vi "7 - Dynamically Rebind Event Handlers.vi"() -> ()   [LabVIEW 2012]
panel:
  out "Slide":dbl(slide) scale=0.0..100.0
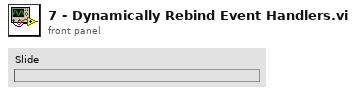
[diagram p1: front panel]
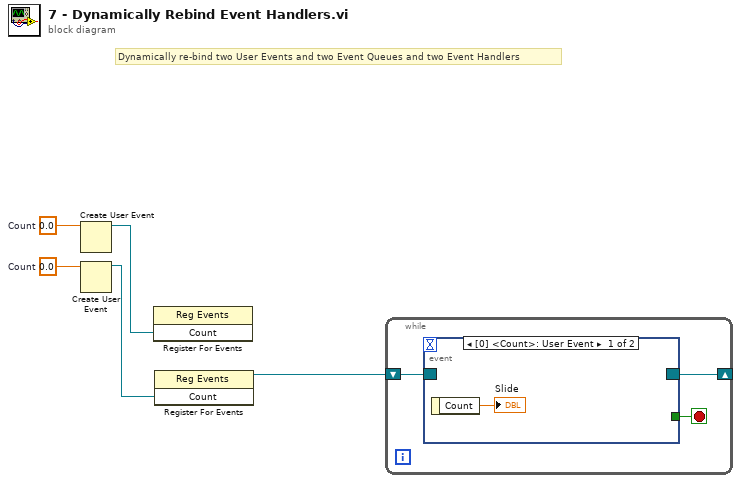
[diagram p0: block diagram]
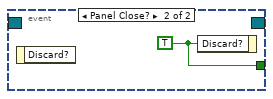
[diagram p2: hidden frame]
diagram:
  w4 = 0.0  # Count
  w5 = 0.0  # Count
  # "Dynamically re-bind two User Events and two Event Queues and two Event Handlers"
  n1 = Create User Event(user event datatype=w5) -> (user event=w3:refnum<user-event>)  [unwired: 1 in, 1 out]
  n2 = Create User Event(user event datatype=w4) -> (user event=w2:refnum<user-event>)  [unwired: 1 in, 1 out]
  n3 = register-events(w3) -> ()  [unwired: 2 in, 2 out]
  n4 = register-events(w2) -> (reference out=w1:refnum<event-registration>)  [unwired: 2 in, 1 out]
  n5 = while {
    shift-right: [w6] -> _
    shift-left: w1 -> [w8]
    stop <- w7 stop-if-true
    n6 = event shown="[0] <Count>: User Event" {
      selector: w8 -> [_ _]
      dyn-events: [_ _] -> w6
      timeout: _ -> [_ _]
      tunnel: [_ w10] -> w7
      event User Event {
        n7 = event-data() -> ("Count"=→"Slide":dbl)  [unwired: 1 in]
      }
      event Panel Close? {
        w10 = TRUE ("Discard?")
        n8 = event-data() -> ()  [unwired: 1 in, 1 out]
        n9 = event-data("Discard?"=w10) -> ()  [unwired: 1 in, 1 out]
      }
    }
  }
